vi "428_TEST_SPEED.vi"() -> ()   [LabVIEW 2016]
panel:
  out "Power":string
  out "millisecond timer value":u32
  out "Wavelength":string="0000.0000\r\n"
  in  "baud rate":u32=921600
  in  "VISA resource name":refnum<visa-resource-name>="COM4"
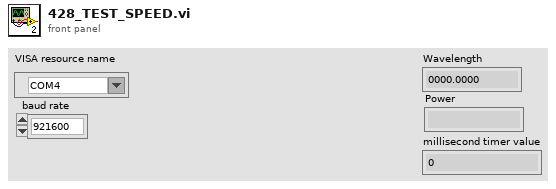
[diagram p1: front panel]
types:
  T1 = enum16{"Power", "Environment", "Wavelength", "Wave Number", "Frequency"}
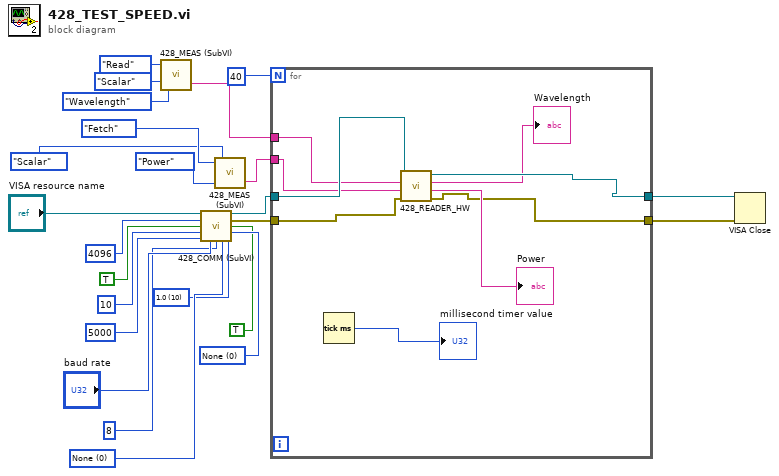
[diagram p0: block diagram]
diagram:
  w17 = u16 0 items=["None", "On"] ("flow control")
  w18 = u16 10 items=["1.0"=10, "1.5"=15, "2.0"=20] ("stop bits")
  w19 = u16 0 items=["None", "Odd", "Even", "Mark", "Space"] ("parity")
  n1 = call "428_MEAS (SubVI).vi"("Measurement Command"=T1."Wavelength", "Response Format"=enum16{"Scalar", "Array"}."Scalar", "Measurement Type"=enum16{"Measure", "Read", "Fetch"}."Read") -> ("String"=w5:string)  [unwired: 1 out]
  n2 = call "428_COMM (SubVI).vi"("VISA resource name"="VISA resource name", "Input\nbuffer size"=u32 4096 ("Input\nbuffer size"), "End read on termination character?"=TRUE, "End write with termination character?"=TRUE, "termination char\n(0xA = '\\n' = LF)"=u8 10 ("termination char\n(0xA = '\\n' = LF)"), "flow control"=w17, "timeout (ms)"=u32 5000, "baud rate"="baud rate", "data bits"=u16 8, "parity"=w19, "stop bits"=w18) -> ("VISA resource name out"=w24:refnum<visa-resource-name>, "error out"=w23:errorcluster)  [unwired: 3 in]
  n3 = call "428_MEAS (SubVI).vi"("Measurement Command"=T1."Power", "Response Format"=enum16{"Scalar", "Array"}."Scalar", "Measurement Type"=enum16{"Measure", "Read", "Fetch"}."Fetch") -> ("String"=w1:string)  [unwired: 1 out]
  n4 = for {
    N: 40 -> [_]
    tunnel: w24 -> [w27]
    tunnel: w23 -> [w28]
    tunnel: [w32] -> w10
    tunnel: [w29] -> w9
    tunnel: w5 -> [w26]
    tunnel: w1 -> [w25]
    n5 = Tick Count (ms)() -> (millisecond timer value=→"millisecond timer value":u32)
    n6 = call "428_READER_HW.vi"("error in (no error)"=w28, "Command 2"=w25, "Command 1"=w26, "VISA resource name"=w27) -> ("error out"=w29:errorcluster, "Power"=→"Power":string, "Wavelength"=→"Wavelength":string, "VISA resource name out"=w32:refnum<visa-resource-name>)  [unwired: 4 in]
  }
  n7 = VISA Close(VISA resource name=w10, error in (no error)=w9) -> ()  [unwired: 1 out]
